vi "Add Or Replace Coord Array.vi"(8 "Coord":cluster{"X":sgl, "Y":sgl}, 9 "Index":i32, 11 "Coord Array In":cluster{"X ":sgl, "Y ":sgl}[](array[cluster])) -> (3 "Coord Array Out":cluster{"X":sgl, "Y":sgl}[](array[cluster]))   [LabVIEW 2013]
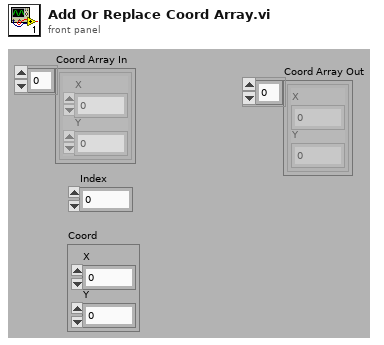
[diagram p1: front panel]
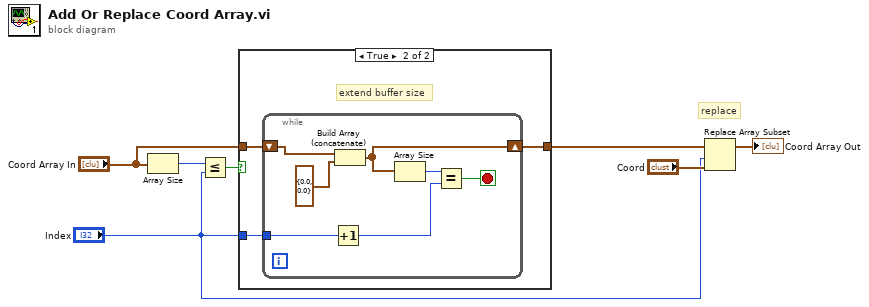
[diagram p0: block diagram]
diagram:
  # "replace"
  n1 = Array Size(array="Coord Array In") -> (size(s)=w7:i32)
  n2 = Less Or Equal?(x=w7, y="Index") -> (x <= y?=w6:bool)
  n3 = case shown="True" w6 {
    tunnel: "Coord Array In" -> [w8 w11]
    tunnel: [w8 w10] -> w4
    tunnel: "Index" -> [_ w9]
    frame False {
    }
    frame True {
      # "extend buffer size"
      n4 = while {
        shift-right: [w16] -> w10
        shift-left: w11 -> [w18]
        tunnel: w9 -> [w14]
        stop <- w13 stop-if-true
        n5 = Increment(x=w14) -> (x+1=w12:i32)
        n6 = Build Array (concatenate)(w18, cluster{"X":sgl, "Y":sgl} {"X"=0.0, "Y"=0.0} ("Centroid Avg")) -> (w16:cluster{"X":sgl, "Y":sgl}[])
        n7 = Array Size(array=w16) -> (size(s)=w15:i32)
        n8 = Equal?(x=w15, y=w12) -> (x = y?=w13:bool)
      }
    }
  }
  n9 = Replace Array Subset(array=w4, new element="Coord", index="Index") -> (→"Coord Array Out":cluster{"X ":sgl, "Y ":sgl}[])
